vi "密码修改（副本）.vi"() -> ()   [LabVIEW 2015]
panel:
  in  "原密码所在位置":path=path "E:/桌面/Desktop/登录测试/user.txt"
  in  "确定修改":bool
  in  "新密码":string
  in  "新账户":string
  in  "密码":string
  in  "账户":string
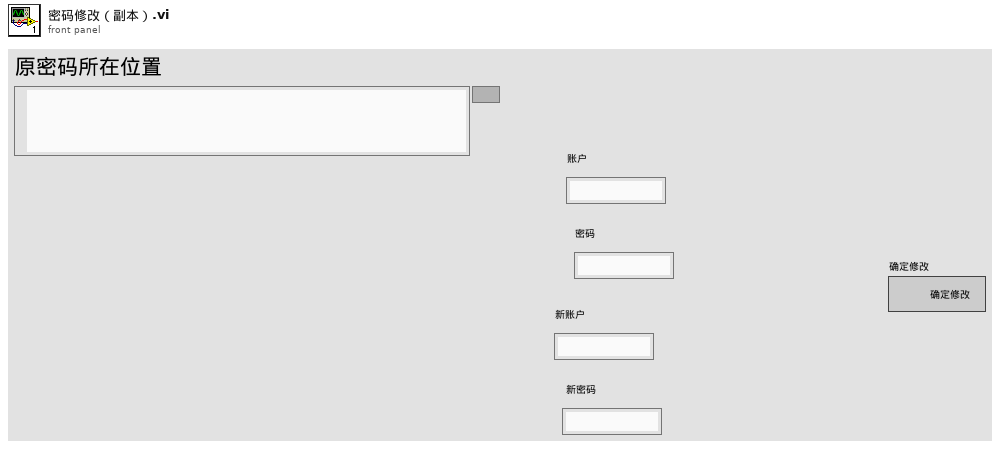
[diagram p1: front panel]
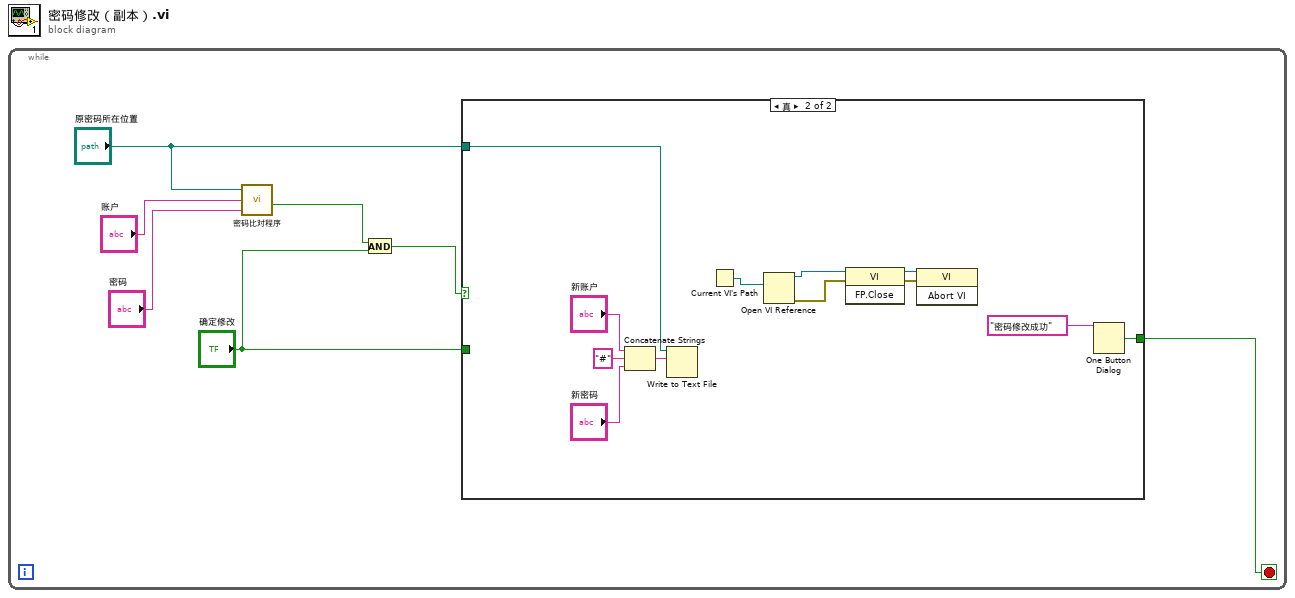
[diagram p0: block diagram]
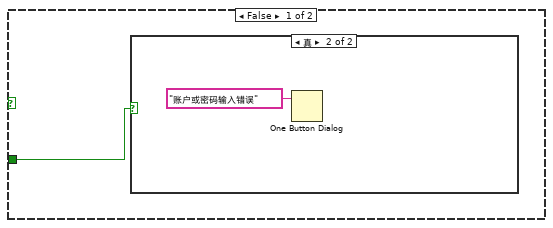
[diagram p2: hidden frame]
diagram:
  n1 = while {
    stop <- w1 stop-if-true
    n2 = call "密码比对程序.vi"("密码"="密码", "账户"="账户", "原密码所在位置"="原密码所在位置") -> ("x = y?"=w5:bool)  [unwired: 5 in]
    n3 = And(x=w5, y="确定修改") -> (x .and. y?=w4:bool)
    n4 = case shown="真" w4 {
      tunnel: "原密码所在位置" -> [_ w17]
      tunnel: "确定修改" -> [w8 _]
      tunnel: [_ w10] -> w1
      frame False {
        n5 = case shown="真" w8 {
          frame False {
          }
          frame True {
            n6 = One Button Dialog(message="账户或密码输入错误" ("消息")) -> ()  [unwired: 1 in, 1 out]
          }
        }
      }
      frame True {
        n7 = Concatenate Strings("新账户", "#" ("字符串"), "新密码") -> (w18:string)
        n8 = Write to Text File(file (use dialog)=w17, text=w18) -> ()  [unwired: 2 in, 3 out]
        n9 = Current VI's Path() -> (path=w13:path)
        n10 = Open VI Reference(vi path=w13) -> (vi reference=w15:refnum<vi>, error out=w14:errorcluster)  [unwired: 5 in]
        n11 = invoke class="VI" method="FP.Close"(reference=w15, error in=w14) -> (reference out=w12:refnum<vi>, error out=w11:errorcluster)  [unwired: 1 in, 1 out]
        n12 = invoke class="VI" method="Abort VI"(reference=w12, error in=w11) -> ()  [unwired: 1 in, 3 out]
        n13 = One Button Dialog(message="密码修改成功" ("消息")) -> (true=w10:bool)  [unwired: 1 in]
      }
    }
  }
